vi "Extract Number String From String.vi"(0 "string":string="123sdaf", 1 "validness":T1(ring), 2 "upper bondary":dbl=360.0, 3 "lower bondary":dbl, 4 "use default":bool, 5 "default":string="0") -> (6 "number string out":string="1.23E+2", 7 "valid input?":bool=TRUE, 8 "Error Messagess":string="No Error")   [LabVIEW 2025]
doc: "Scan any string for a number, beginning at the input index. Any of the following formats are recognized:\n123 1.23 1.23e2 1.23E2\nNo spaces or other characters may appear within the number, but any characters may appear before or after the number. Returns true if a number is found, the value of the number, and the index of the first character after the number.\nScott Hannahs, FBNML 1991"
uses:
  <vilib>/Utility/error.llb/Trim Whitespace One-Sided.vi
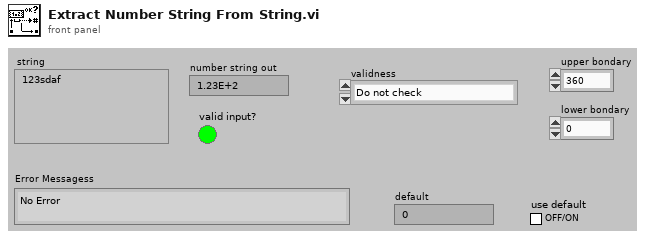
[diagram p1: front panel]
types:
  T1 = enum16{"Do not check", "Larger than 0", "Positive", "Upper and Lower bondaries", "Negative", "Boolean"}
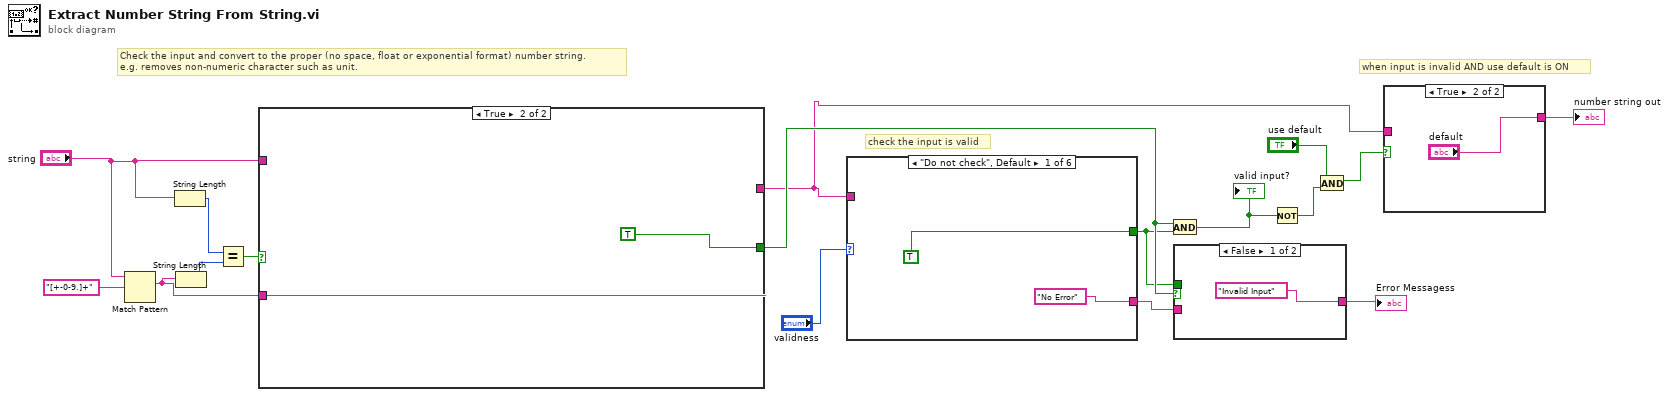
[diagram p0: block diagram]
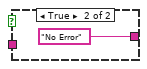
[diagram p4: hidden frame]
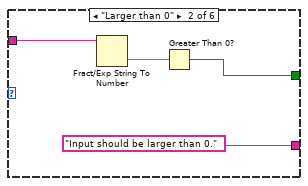
[diagram p5: hidden frame]
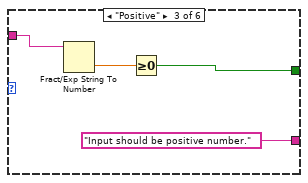
[diagram p6: hidden frame]
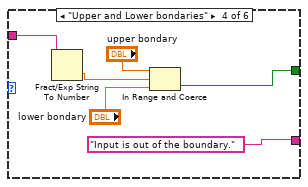
[diagram p7: hidden frame]
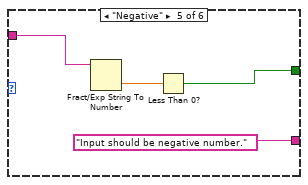
[diagram p8: hidden frame]
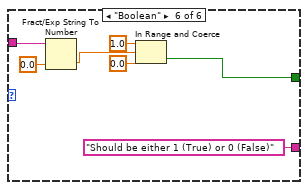
[diagram p9: hidden frame]
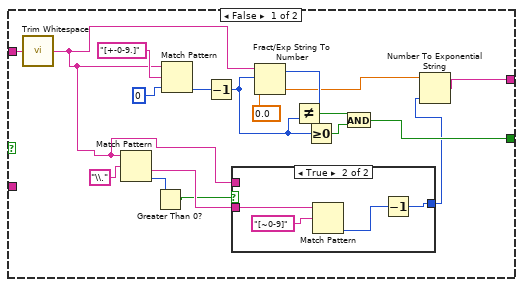
[diagram p10: hidden frame]
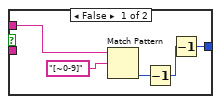
[diagram p11: hidden frame]
diagram:
  # "check the input is valid"
  # "Check the input and convert to the proper (no space, float or exponential format) number string.\ne.g. removes non-numeric character such as unit."
  # "when input is invalid AND use default is ON"
  n1 = Match Pattern(string="string", regular expression="[+-0-9.]+") -> (match substring=w12:string)  [unwired: 1 in, 3 out]
  n2 = String Length(string="string") -> (length=w16:i32)
  n3 = String Length(string=w12) -> (length=w15:i32)
  n4 = Equal?(x=w16, y=w15) -> (x = y?=w14:bool)
  n5 = case shown="True" w14 {
    tunnel: "string" -> [w23 _]
    tunnel: w12 -> [_ w46]
    tunnel: [w35 w46] -> w1
    tunnel: [w25 TRUE] -> w10
    frame False {
      n6 = call <vilib>:"Trim Whitespace.vi"("string"=w23) -> ("trimmed string"=w18:string)  [unwired: 1 in]
      n7 = Match Pattern(string=w18, regular expression="\\.") -> (after substring=w21:string, offset past match=w20:i32)  [unwired: 1 in, 2 out]
      n8 = Greater Than 0?(x=w20) -> (x > 0?=w19:bool)
      n9 = Match Pattern(string=w18, regular expression="[+-0-9.]", offset (0)=0) -> (offset past match=w33:i32)  [unwired: 3 out]
      n10 = Decrement(x=w33) -> (x-1=w31:i32)
      n11 = case shown="True" w19 {
        tunnel: [w36 w41] -> w22
        tunnel: w21 -> [_ w42]
        tunnel: w18 -> [w39 _]
        frame False {
          n12 = Match Pattern(string=w39, regular expression="[~0-9]") -> (offset past match=w38:i32)  [unwired: 1 in, 3 out]
          n13 = Decrement(x=w38) -> (x-1=w37:i32)
          n14 = Decrement(x=w37) -> (x-1=w36:i32)
        }
        frame True {
          n15 = Match Pattern(string=w42, regular expression="[~0-9]") -> (offset past match=w43:i32)  [unwired: 1 in, 3 out]
          n16 = Decrement(x=w43) -> (x-1=w41:i32)
        }
      }
      n17 = Fract/Exp String To Number(string=w18, offset=w31, default (0 dbl)=0.0) -> (offset past number=w30:i32, number=w26:dbl)  [unwired: 1 in]
      n18 = Not Equal?(x=w30, y=w31) -> (x != y?=w29:bool)
      n19 = Greater Or Equal To 0?(x=w31) -> (x >= 0?=w28:bool)
      n20 = And(x=w29, y=w28) -> (x .and. y?=w25:bool)
      n21 = Number To Exponential String(number=w26, precision (6)=w22) -> (E-format string=w35:string)  [unwired: 2 in]
    }
    frame True {
    }
  }
  n22 = case shown="\"Do not check\", Default" "validness" {
    tunnel: w1 -> [_ w52 w55 w62 w65 w73]
    tunnel: [TRUE ("y") w50 w54 w58 w64 w68] -> w8
    tunnel: ["No Error" ("Error Messagess") "Input should be larger than 0." ("Error Messagess") "Input should be positive number." ("Error Messagess") "Input is out of the boundary." ("Error Messagess") "Input should be negative number." ("Error Messagess") "Should be either 1 (True) or 0 (False)" ("Error Messagess")] -> w9
    frame "Do not check", Default {
    }
    frame "Larger than 0" {
      n23 = Fract/Exp String To Number(string=w52) -> (number=w51:dbl)  [unwired: 3 in, 1 out]
      n24 = Greater Than 0?(x=w51) -> (x > 0?=w50:bool)
    }
    frame "Positive" {
      n25 = Fract/Exp String To Number(string=w55) -> (number=w56:dbl)  [unwired: 3 in, 1 out]
      n26 = Greater Or Equal To 0?(x=w56) -> (x >= 0?=w54:bool)
    }
    frame "Upper and Lower bondaries" {
      n27 = Fract/Exp String To Number(string=w62) -> (number=w61:dbl)  [unwired: 3 in, 1 out]
      n28 = In Range and Coerce(upper limit="upper bondary", x=w61, lower limit="lower bondary") -> (In Range?=w58:bool)  [unwired: 1 out]
    }
    frame "Negative" {
      n29 = Fract/Exp String To Number(string=w65) -> (number=w66:dbl)  [unwired: 3 in, 1 out]
      n30 = Less Than 0?(x=w66) -> (x < 0?=w64:bool)
    }
    frame "Boolean" {
      n31 = Fract/Exp String To Number(string=w73, default (0 dbl)=0.0 ("default (0 DBL)")) -> (number=w71:dbl)  [unwired: 2 in, 1 out]
      n32 = In Range and Coerce(upper limit=1.0, x=w71, lower limit=0.0) -> (In Range?=w68:bool)  [unwired: 1 out]
    }
  }
  n33 = And(x=w10, y=w8) -> (x .and. y?=w6:bool)
  "valid input?" <- w6
  n34 = case shown="False" w10 {
    tunnel: ["Invalid Input" ("Error Messagess") w76] -> w7
    tunnel: w9 -> [_ w75]
    tunnel: w8 -> [_ w77]
    frame False {
    }
    frame True {
      n35 = case shown="False" w77 {
        tunnel: [w78 "No Error" ("Error Messagess")] -> w76
        tunnel: w75 -> [w78 _]
        frame False {
        }
        frame True {
        }
      }
    }
  }
  "Error Messagess" <- w7
  n36 = Not(x=w6) -> (.not. x?=w5:bool)
  n37 = And(x="use default", y=w5) -> (x .and. y?=w3:bool)
  n38 = case shown="True" w3 {
    tunnel: [w80 "default"] -> w2
    tunnel: w1 -> [w80 _]
    frame False {
    }
    frame True {
    }
  }
  "number string out" <- w2
